vi "Main.vi"() -> ()   [LabVIEW 2019, in "Personalities Tool.lvlib"]
uses:
  Personalities Tool.lvlib
  Controls/QMH Data.ctl
  Controls/Personality Type.ctl
  Controls/roboRIO Connection Information.ctl
  Controls/Diff Key.ctl
  subVIs/Message Queue/Enqueue Message (Single).vi
panel:
  out "Personality":string
  out "Status":string
  in  "File editor":string
  in  "Download personality to RIO":bool
  in  "Save personality locally":bool
  in  "Connect":bool
  in  "Open local personality":bool
  in  "Stop":bool
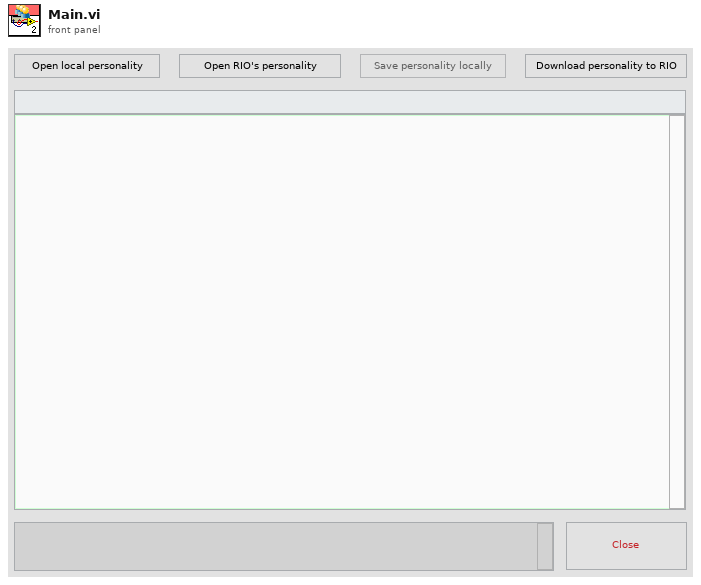
[diagram p1: front panel]
types:
  T1 = typedef "Personalities Tool.lvlib/QMH Data.ctl" = cluster{"Status":string, "Open Personality File Path":path, "File text":string, "Selected Personality":T2, "roboRIO Connection Information":T3, "VI reference":refnum<vi>, "Save personality locally reference":refnum<vi>, "File editor reference":refnum<vi>}
  T2 = typedef "Personalities Tool.lvlib/Personality Type.ctl" = cluster{"Valid personality?":bool, "Personality":string}
  T3 = typedef "Personalities Tool.lvlib/roboRIO Connection Information.ctl" = cluster{"Connected?":bool, "IP Address":string, "SN":string, "Personality":T2, "Name":string}
  T4 = typedef "Personalities Tool.lvlib/All Message Queues.ctl" = cluster{"UI":refnum<queue>}
  T5 = enum8{"Enabled", "Disabled", "Disabled and Grayed Out"}
  T6 = typedef "Personalities Tool.lvlib/Diff Key.ctl" = cluster{"Section":string, "Local":variant, "roboRIO":variant, "Selection":enum32{"Item 0", "Item 1"}, "Key":string}
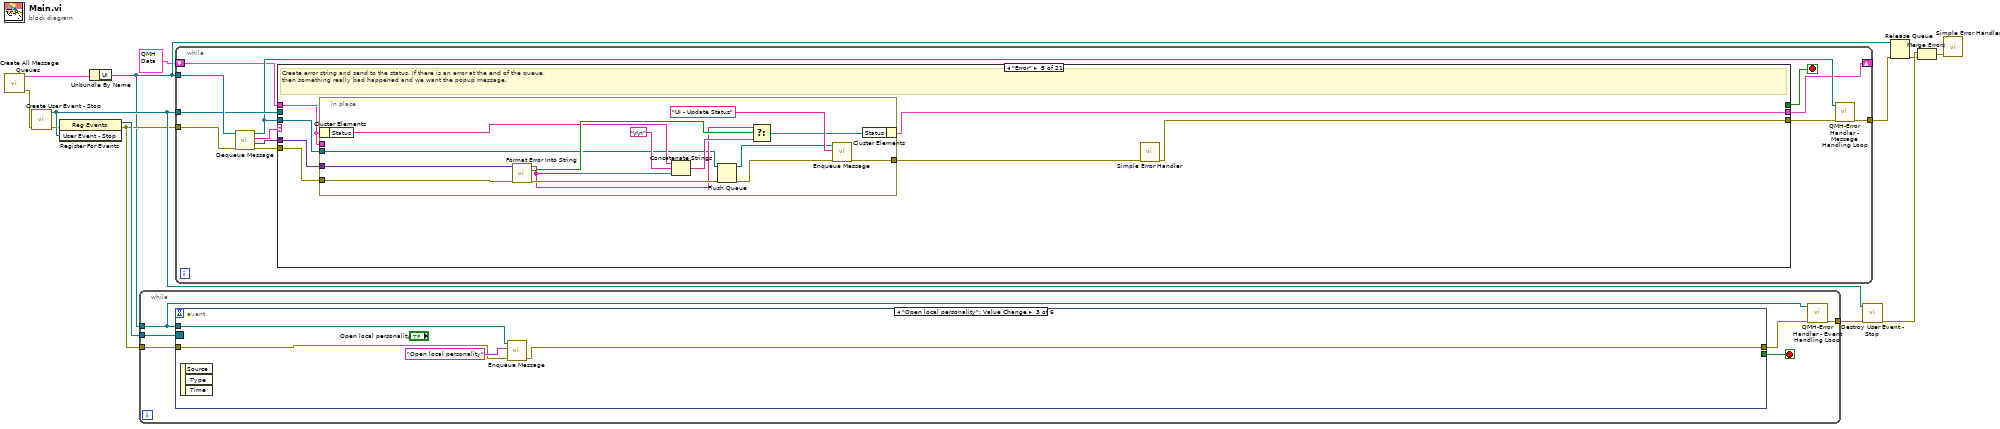
[diagram p0: block diagram]
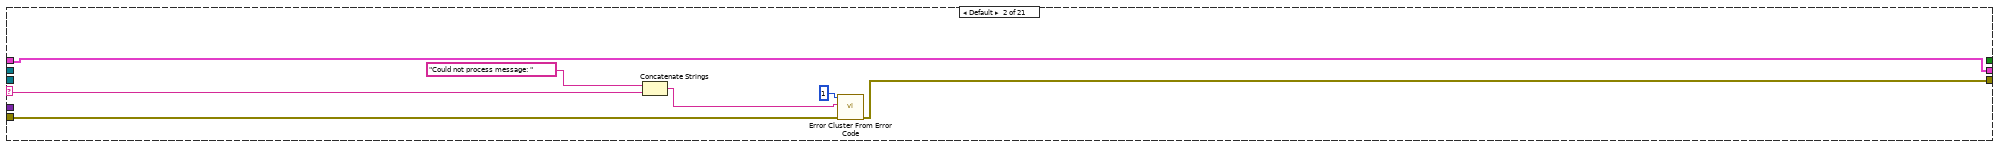
[diagram p3: hidden frame]
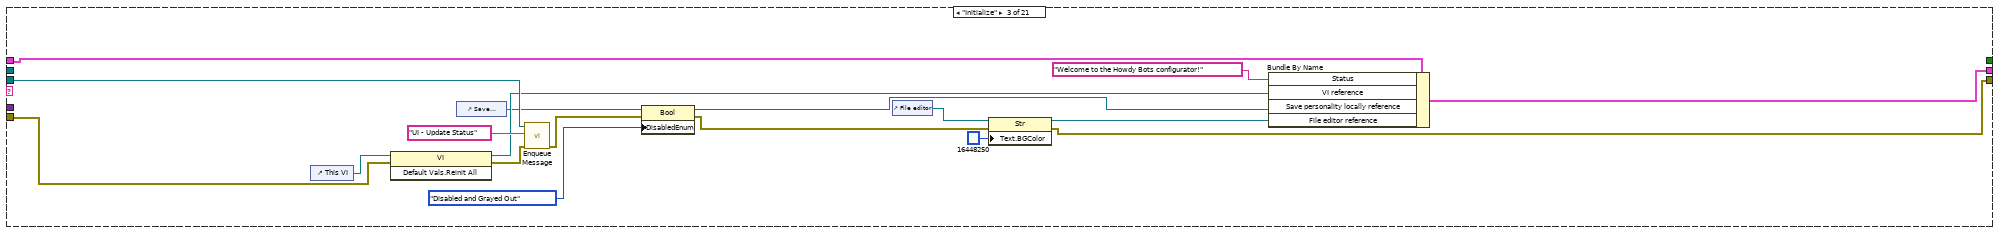
[diagram p4: hidden frame]
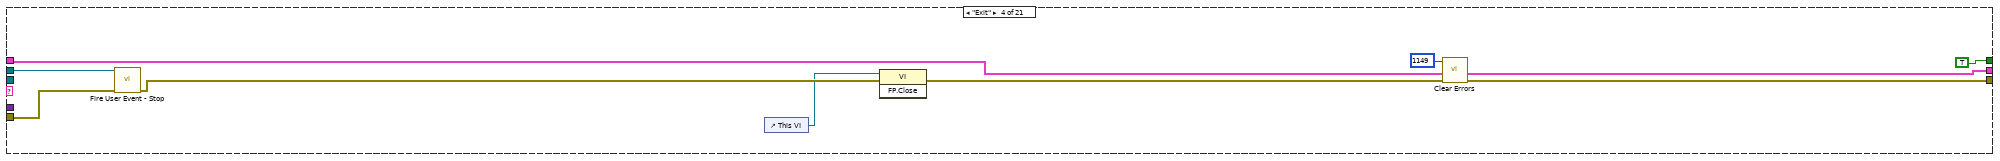
[diagram p5: hidden frame]
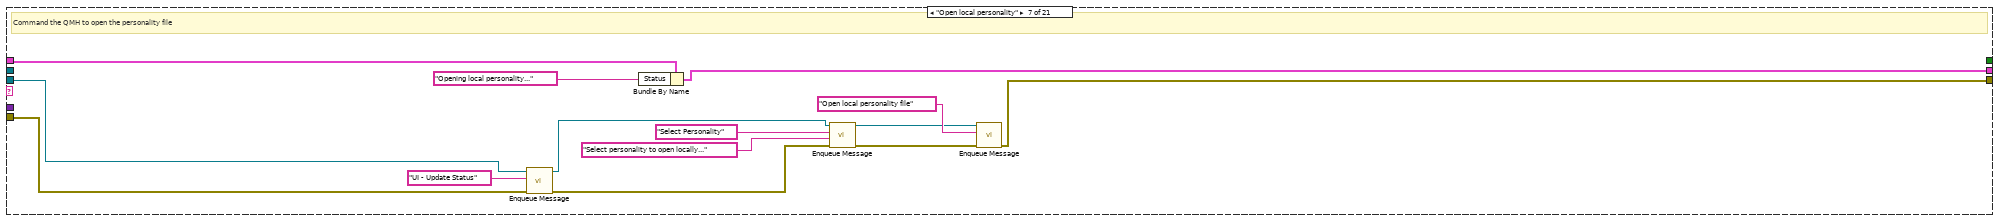
[diagram p7: hidden frame]
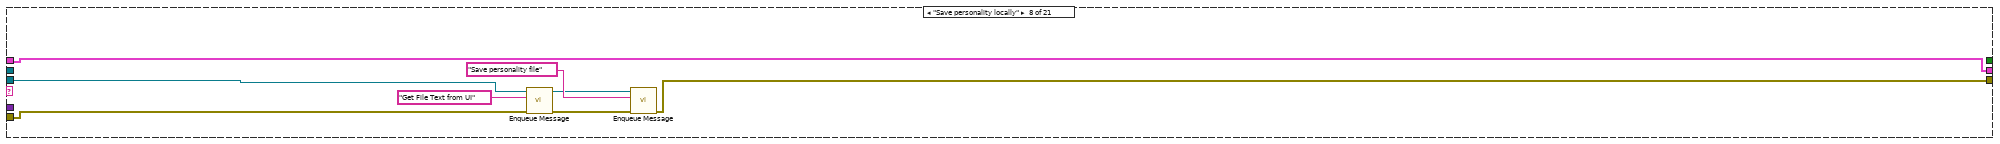
[diagram p8: hidden frame]
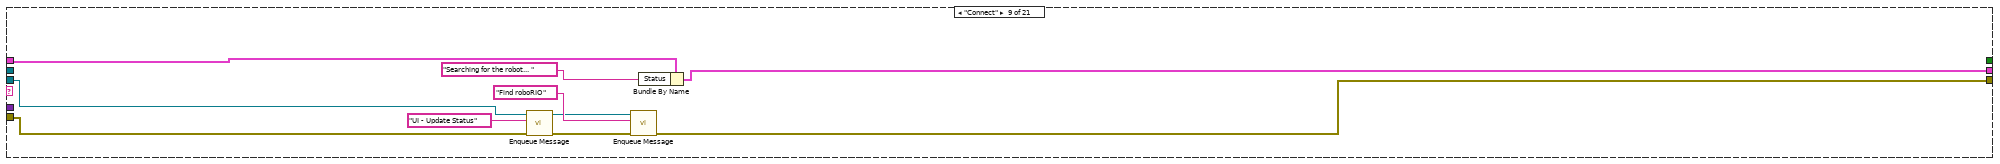
[diagram p9: hidden frame]
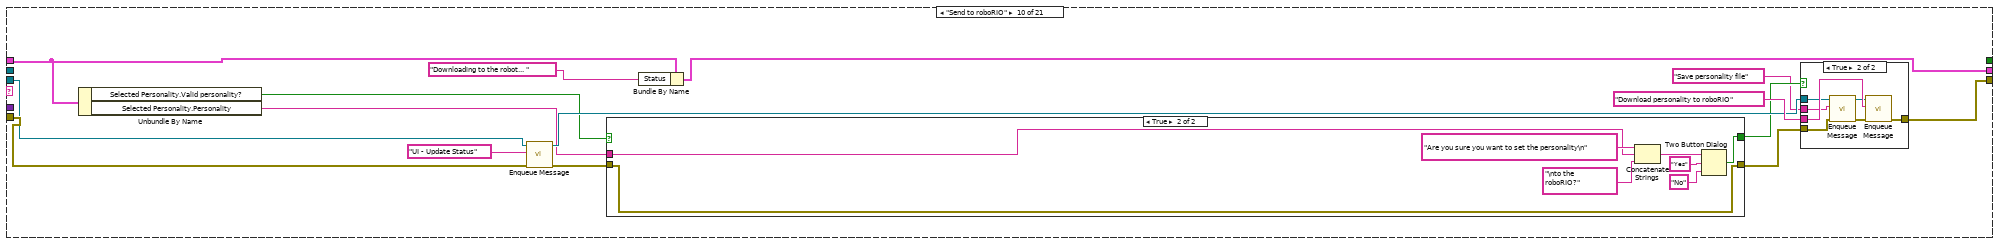
[diagram p10: hidden frame]
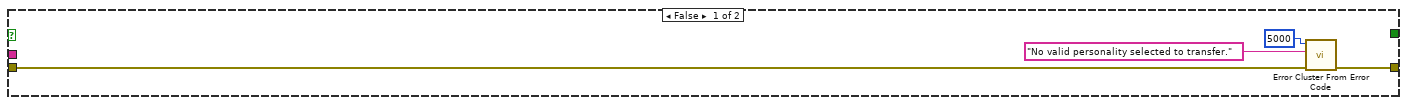
[diagram p11: hidden frame]
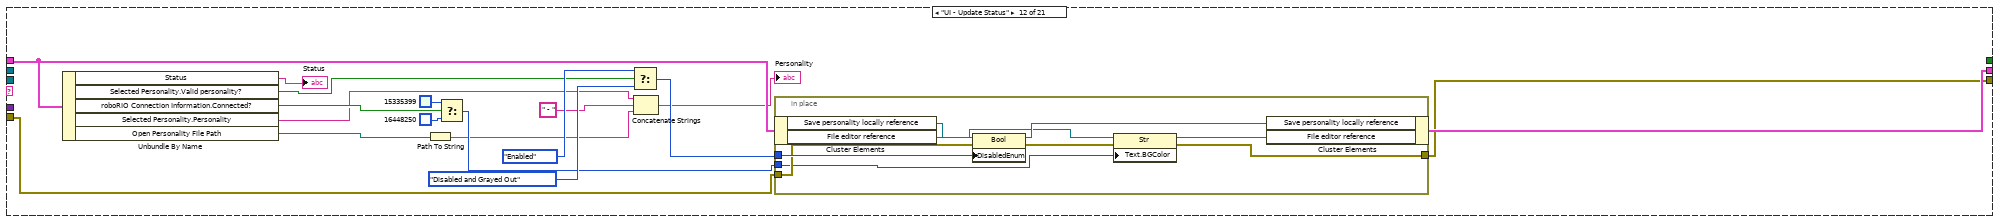
[diagram p14: hidden frame]
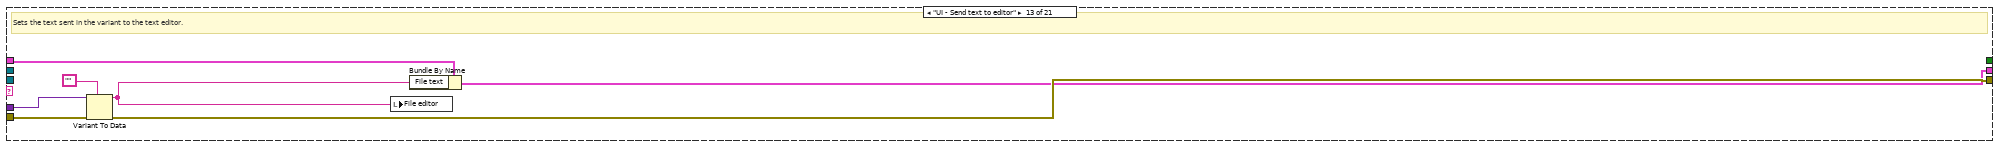
[diagram p15: hidden frame]
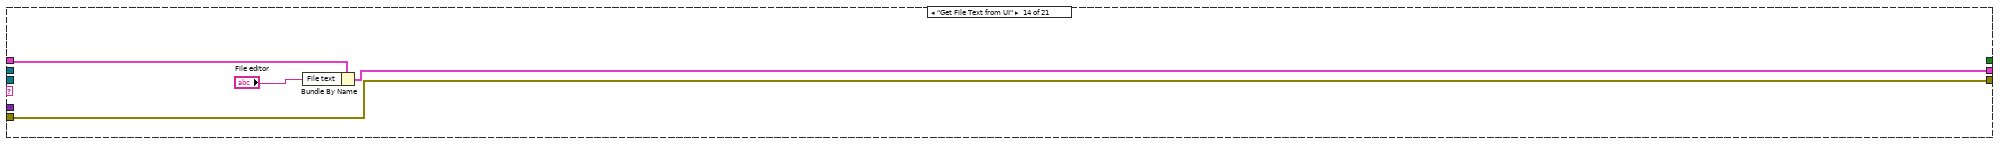
[diagram p16: hidden frame]
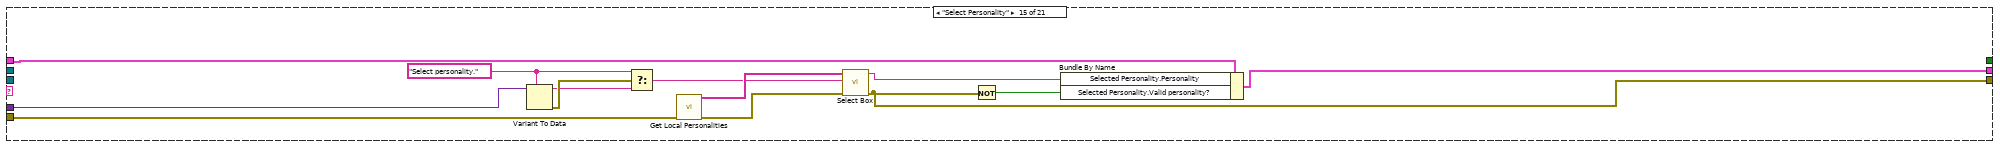
[diagram p17: hidden frame]
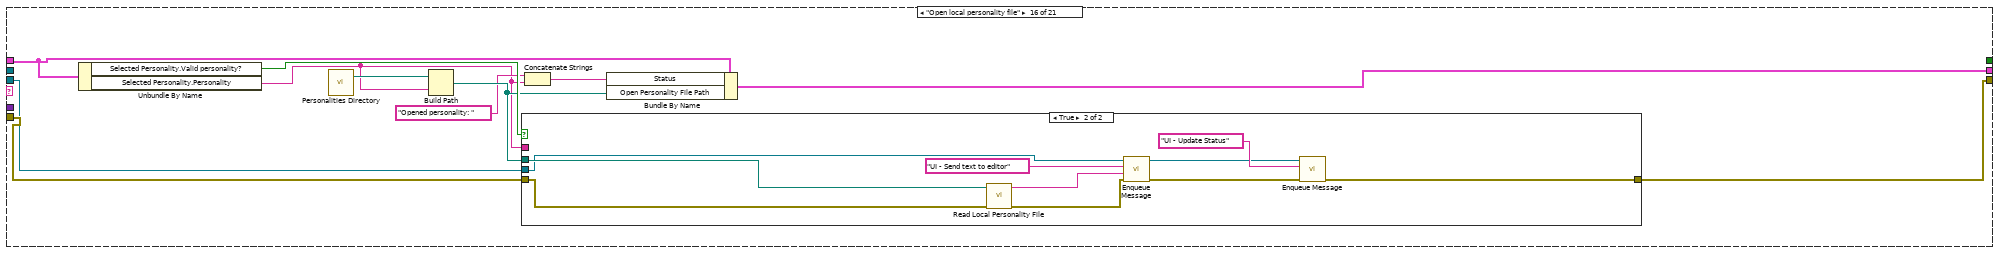
[diagram p18: hidden frame]
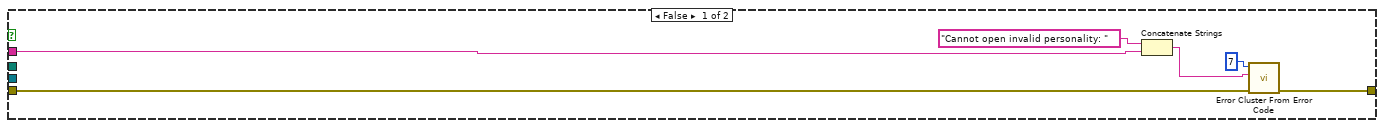
[diagram p19: hidden frame]
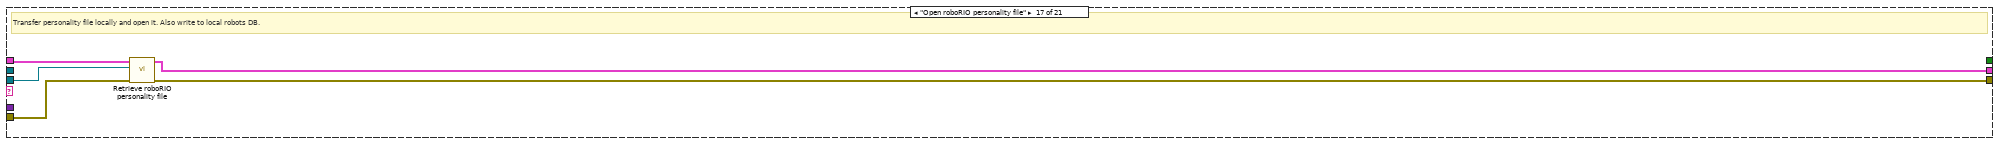
[diagram p20: hidden frame]
diagram:
  n1 = call "Create All Message Queues.vi"() -> ("error out"=w10:errorcluster, "Message Queues out"=w11:T4)  [unwired: 10 in]
  n2 = call "Create User Event - Stop.vi"("error in (no error)"=w10) -> ("error out"=w9:errorcluster, "User Event - Stop"=w12:refnum<user-event>)  [unwired: 9 in]
  n3 = register-events(error in=w9, w12) -> (reference out=w13:refnum<event-registration>, error out=w8:errorcluster)  [unwired: 1 in]
  n4 = Unbundle By Name(w11) -> ("UI"=w4:refnum<queue>)
  n5 = while {
    tunnel: w13 -> [w19]
    tunnel: w4 -> [w14]
    tunnel: w8 -> [w18]
    tunnel: [w15] -> w7
    stop <- w17 stop-if-true
    n6 = event shown="[2] \"Open local personality\": Value Change" {
      selector: w19 -> [_ _ _ _ _ _]
      dyn-events: _ -> [_ _ _ _ _ _]
      timeout: _ -> [_ _ _ _ _ _]
      tunnel: w14 -> [_ w22 w37 w41 w45 w52]
      tunnel: w18 -> [w20 w24 w39 w43 w47 w50]
      tunnel: [TRUE _ _ _ _ _] -> w17
      tunnel: [w20 w27 w38 w42 w46 w54] -> w16
      event User Event {
        n7 = event-data() -> ()  [unwired: 1 in, 3 out]
      }
      event "Stop": Value Change; Panel Close {
        n8 = event-data() -> ()  [unwired: 1 in, 3 out]
        n9 = disable-structure shown="Enabled" {
          disable-tunnel: [w28 _] -> w25
          frame Disabled {
            n10 = Two Button Dialog(message="Save opened personality before closing?", 1:"No" ("F button name (\"Cancel\")"), 2:"Yes" ("T button name (\"OK\")")) -> (T button?=w28:bool)
          }
          frame Enabled {
            # "Disabled saving check to ensure we do not accidentally override the\nfile with constants and introduce typos"
          }
        }
        n11 = case shown="True" w25 {
          tunnel: [w32 w34] -> w23
          tunnel: w24 -> [w32 w35]
          tunnel: w22 -> [_ w33]
          frame False {
          }
          frame True {
            n12 = call-poly "Enqueue Message.vi"("error in (no error)"=w35, "Message"="Save personality locally", "Message Queue"=w33) -> ("error out"=w34:errorcluster)  [unwired: 7 in, 1 out]
          }
        }
        n13 = call-poly "Enqueue Message.vi"("error in (no error)"=w23, "Message"="Exit", "Message Queue"=w22) -> ("error out"=w27:errorcluster)  [unwired: 7 in, 1 out]
      }
      event "Open local personality": Value Change {
        n14 = event-data() -> ()  [unwired: 1 in, 3 out]
        n15 = call-poly "Enqueue Message.vi"("error in (no error)"=w39, "Message"="Open local personality", "Message Queue"=w37) -> ("error out"=w38:errorcluster)  [unwired: 7 in, 1 out]
      }
      event "Connect": Value Change {
        n16 = event-data() -> ()  [unwired: 1 in, 3 out]
        n17 = call-poly "Enqueue Message.vi"("error in (no error)"=w43, "Message"="Connect", "Message Queue"=w41) -> ("error out"=w42:errorcluster)  [unwired: 7 in, 1 out]
      }
      event "Save personality locally": Value Change {
        n18 = event-data() -> ()  [unwired: 1 in, 3 out]
        n19 = call-poly "Enqueue Message.vi"("error in (no error)"=w47, "Message"="Save personality locally", "Message Queue"=w45) -> ("error out"=w46:errorcluster)  [unwired: 7 in, 1 out]
      }
      event "Download personality to RIO": Value Change {
        n20 = event-data() -> ()  [unwired: 1 in, 3 out]
        n21 = call-poly "Enqueue Message.vi"("error in (no error)"=w50, "Message"="Save personality locally", "Message Queue"=w52) -> ("error out"=w49:errorcluster, "dup Message Queue"=w51:refnum<queue>)  [unwired: 7 in]
        n22 = call-poly "Enqueue Message.vi"("error in (no error)"=w49, "Message"="Send to roboRIO", "Message Queue"=w51) -> ("error out"=w54:errorcluster)  [unwired: 7 in, 1 out]
      }
    }
    n23 = call "QMH-Error Handler - Event Handling Loop.vi"("error in (no error)"=w16, "Message Queue"=w14) -> ("dup error in"=w15:errorcluster)  [unwired: 8 in, 1 out]
  }
  n24 = while {
    tunnel: w12 -> [w60]
    tunnel: w4 -> [w67]
    tunnel: w8 -> [w66]
    tunnel: [w61] -> w5
    shift-right: [w57] -> _
    shift-left: T1 {"Status"="", "Open Personality File Path"=path "", "File text"="", "Selected Personality"={"Valid personality?"=FALSE, "Personality"=""}, "roboRIO Connection Information"={"Connected?"=FALSE, "IP Address"="", "SN"="", "Personality"={"Valid personality?"=FALSE, "Personality"=""}, "Name"=""}, "VI reference"=refnum, "Save personality locally reference"=refnum, "File editor reference"=refnum} ("UI Data") -> [w56]
    stop <- w58 stop-if-true
    n25 = call "Dequeue Message.vi"("error in (no error)"=w66, "Message Queue"=w67) -> ("error out"=w64:errorcluster, "Message Data"=w63:variant, "Message"=w65:string, "dup Message Queue"=w59:refnum<queue>)  [unwired: 6 in]
    n26 = case shown="\"Error\"" w65 {
      selector: w65 -> [_ w71 _ _ _ _ _ _ _ _ _ _ _ _ _ _ _ _ _ _ _]
      tunnel: w64 -> [w68 w76 w87 w103 w110 w125 w137 w143 w153 w170 w194 w205 w228 w232 w241 w255 w277 w287 w313 w330 w352]
      tunnel: [w68 w75 w80 w96 w106 w125 w128 w141 w151 w168 w194 w206 w227 w232 w243 w253 w278 w285 w314 w316 w349] -> w62
      tunnel: w63 -> [_ _ _ _ w109 _ _ _ _ _ _ _ w226 _ w238 _ _ _ _ _ w351]
      tunnel: w59 -> [_ _ w90 _ w108 _ w138 w142 w152 w169 _ _ _ _ _ w250 w274 w284 w311 w318 w343]
      tunnel: w60 -> [_ _ _ w102 _ _ _ _ _ _ _ _ _ _ _ _ _ _ _ _ _]
      tunnel: [_ _ _ TRUE _ _ _ _ _ _ _ _ _ _ _ _ _ _ _ _ _] -> w58
      tunnel: [w69 w70 w93 w99 w104 w126 w136 w148 w150 w167 w195 w211 w224 w231 w245 w256 w276 w288 w315 w324 w347] -> w57
      tunnel: w56 -> [w69 w70 w94 w99 w105 w126 w140 w148 w158 w164 w195 w212 w229 w233 w246 w257 w275 w289 w312 w329 w344]
      frame "---BASE QMH MESSAGES---" {
        # "This case must not execute ever, used just for documentation"
      }
      frame Default {
        n27 = Concatenate Strings("Could not process message: " ("error message (\"\")"), w71) -> (w72:string)
        n28 = call <vilib>:"Error Cluster From Error Code.vi"("error in (no error)"=w76, "error message (\"\")"=w72, "error code (0)"=1) -> ("error out"=w75:errorcluster)  [unwired: 6 in]
      }
      frame "Initialize" {
        n29 = control-ref of="This VI"() -> (w88:refnum<vi>)
        n30 = invoke class="VI" method="Default Vals.Reinit All"(reference=w88, error in=w87) -> (reference out=w85:refnum<vi>, error out=w86:errorcluster)  [unwired: 1 in, 1 out]
        n31 = control-ref of="Save personality locally"() -> (w83:refnum<vi>)
        n32 = call-poly "Enqueue Message.vi"("error in (no error)"=w86, "Message"="UI - Update Status", "Message Queue"=w90) -> ("error out"=w89:errorcluster)  [unwired: 7 in, 1 out]
        n33 = property class="Bool"(reference=w83, error in=w89, "DisabledEnum"=T5."Disabled and Grayed Out" ("Disabled")) -> (reference out=w82:refnum<vi>, error out=w84:errorcluster)
        n34 = control-ref of="File editor"() -> (w79:refnum<vi>)
        n35 = property class="Str"(reference=w79, error in=w84, "Text.BGColor"=u32 16448250 ("Text.Colors:BG Color")) -> (reference out=w78:refnum<vi>, error out=w80:errorcluster)
        n36 = Bundle By Name(cluster=w94, "Status"="Welcome to the Howdy Bots configurator!" ("element"), "VI reference"=w85, "Save personality locally reference"=w82, "File editor reference"=w78) -> (w93:T1)
      }
      frame "Exit" {
        n37 = call "Fire User Event - Stop.vi"("error in (no error)"=w103, "User Event - Stop"=w102) -> ("error out"=w101:errorcluster)  [unwired: 9 in]
        n38 = control-ref of="This VI"() -> (w97:refnum<vi>)
        n39 = invoke class="VI" method="FP.Close"(reference=w97, error in=w101) -> (error out=w98:errorcluster)  [unwired: 1 in, 2 out]
        n40 = call <vilib>:"Clear Errors.vi"("error in (no error)"=w98, "specific error code to clear (0: all)"=1149) -> ("error out"=w96:errorcluster)  [unwired: 4 in, 1 out]
      }
      frame "Error" {
        # "Create error string and send to the status. If there is an error at the end of the queue, \nthen something really bad happened and we want the popup message."
        n41 = in-place {
          in-place-border: w110 -> [w124]
          in-place-border: w109 -> [w123]
          in-place-border: w108 -> [w112]
          in-place-border: [w121] -> w107
          in-place-border: w105 -> [_]
          n42 = in-place-cluster #1(w105) -> ("Status"=w115:string)
          n43 = call "Format Error Into String.vi"("error in (no error)"=w124, "Message Data"=w123) -> ("error out"=w120:errorcluster, "error?"=w119:bool, "message"=w117:string)  [unwired: 7 in]
          n44 = Concatenate Strings(w115, "\r\n", w117) -> (w118:string)
          n45 = Flush Queue(queue=w112, error in (no error)=w120) -> (queue out=w111:refnum<queue>, error out=w113:errorcluster)  [unwired: 1 out]
          n46 = Select(t=w117, s=w119, f=w118) -> (s? t:f=w114:string)
          n47 = call-poly "Enqueue Message.vi"("error in (no error)"=w113, "Message"="UI - Update Status", "Message Queue"=w111) -> ("error out"=w121:errorcluster)  [unwired: 7 in, 1 out]
          n48 = in-place-cluster #1("Status"=w114) -> (w104:T1)
        }
        n49 = call <vilib>:"Simple Error Handler.vi"("error in (no error)"=w107) -> ("error out"=w106:errorcluster)  [unwired: 4 in, 4 out]
      }
      frame "---UI MESSAGES---" {
        # "This case must not execute ever, used just for documentation"
      }
      frame "Open local personality" {
        # "Command the QMH to open the personality file"
        n50 = call-poly "Enqueue Message.vi"("error in (no error)"=w137, "Message"="UI - Update Status", "Message Queue"=w138) -> ("error out"=w132:errorcluster, "dup Message Queue"=w133:refnum<queue>)  [unwired: 7 in]
        n51 = Bundle By Name(cluster=w140, "Status"="Opening local personality...") -> (w136:T1)
        n52 = call-poly "Enqueue Message.vi"("error in (no error)"=w132, "Message Data"="Select personality to open locally..." ("Message"), "Message"="Select Personality", "Message Queue"=w133) -> ("error out"=w129:errorcluster, "dup Message Queue"=w127:refnum<queue>)  [unwired: 6 in]
        n53 = call-poly "Enqueue Message.vi"("error in (no error)"=w129, "Message"="Open local personality file", "Message Queue"=w127) -> ("error out"=w128:errorcluster)  [unwired: 7 in, 1 out]
      }
      frame "Save personality locally" {
        n54 = call-poly "Enqueue Message.vi"("error in (no error)"=w143, "Message"="Get File Text from UI", "Message Queue"=w142) -> ("error out"=w144:errorcluster, "dup Message Queue"=w145:refnum<queue>)  [unwired: 7 in]
        n55 = call-poly "Enqueue Message.vi"("error in (no error)"=w144, "Message"="Save personality file", "Message Queue"=w145) -> ("error out"=w141:errorcluster)  [unwired: 7 in, 1 out]
      }
      frame "Connect" {
        n56 = call-poly "Enqueue Message.vi"("error in (no error)"=w153, "Message"="UI - Update Status", "Message Queue"=w152) -> ("error out"=w154:errorcluster, "dup Message Queue"=w155:refnum<queue>)  [unwired: 7 in]
        n57 = call-poly "Enqueue Message.vi"("error in (no error)"=w154, "Message"="Find roboRIO", "Message Queue"=w155) -> ("error out"=w151:errorcluster)  [unwired: 7 in, 1 out]
        n58 = Bundle By Name(cluster=w158, "Status"="Searching for the robot... ") -> (w150:T1)
      }
      frame "Send to roboRIO" {
        n59 = Unbundle By Name(w164) -> ("Selected Personality.Valid personality?"=w162:bool, "Selected Personality.Personality"=w163:string)
        n60 = call-poly "Enqueue Message.vi"("error in (no error)"=w170, "Message"="UI - Update Status", "Message Queue"=w169) -> ("error out"=w161:errorcluster, "dup Message Queue"=w171:refnum<queue>)  [unwired: 7 in]
        n61 = case shown="True" w162 {
          tunnel: [_ w182] -> w165
          tunnel: w163 -> [_ w179]
          tunnel: [w176 w178] -> w160
          tunnel: w161 -> [w177 w178]
          frame False {
            n62 = call <vilib>:"Error Cluster From Error Code.vi"("error in (no error)"=w177, "error message (\"\")"="No valid personality selected to transfer." ("error message (\"\")"), "error code (0)"=5000) -> ("error out"=w176:errorcluster)  [unwired: 6 in]
          }
          frame True {
            n63 = Concatenate Strings("Are you sure you want to set the personality\n" ("message"), w179, "\nto the roboRIO?" ("message")) -> (w181:string)
            n64 = Two Button Dialog(message=w181, 1:"No" ("F button name (\"Cancel\")"), 2:"Yes" ("T button name (\"OK\")")) -> (T button?=w182:bool)
          }
        }
        n65 = Bundle By Name(cluster=w164, "Status"="Downloading to the robot... ") -> (w167:T1)
        n66 = case shown="True" w165 {
          tunnel: "Download personality to roboRIO" ("Message") -> [_ w193]
          tunnel: w171 -> [_ w189]
          tunnel: w160 -> [w186 w192]
          tunnel: [w186 w190] -> w168
          tunnel: "Save personality file" ("Message") -> [_ w187]
          frame False {
          }
          frame True {
            n67 = call-poly "Enqueue Message.vi"("error in (no error)"=w192, "Message"=w187, "Message Queue"=w189) -> ("error out"=w191:errorcluster, "dup Message Queue"=w188:refnum<queue>)  [unwired: 7 in]
            n68 = call-poly "Enqueue Message.vi"("error in (no error)"=w191, "Message"=w193, "Message Queue"=w188) -> ("error out"=w190:errorcluster)  [unwired: 7 in, 1 out]
          }
        }
      }
      frame "---SUPPORT FUNCTIONS---" {
        # "This case must not execute ever, used just for documentation"
      }
      frame "UI - Update Status" {
        n69 = Unbundle By Name(w212) -> ("Status"=→"Status":string, "Selected Personality.Valid personality?"=w208:bool, "roboRIO Connection Information.Connected?"=w204:bool, "Selected Personality.Personality"=w199:string, "Open Personality File Path"=w200:path)
        n70 = Path To String(path=w200) -> (string=w198:string)
        n71 = Select(t=u32 15335399 ("Text.Colors:FG Color"), s=w204, f=u32 16448250 ("Text.Colors:BG Color")) -> (s? t:f=w203:u32)
        n72 = Select(t=T5."Enabled" ("Disabled"), s=w208, f=T5."Disabled and Grayed Out" ("Disabled")) -> (s? t:f=w209:T5)
        n73 = Concatenate Strings(w199, " - " ("string"), w198) -> (→"Personality":string)
        n74 = in-place {
          in-place-border: w209 -> [w222]
          in-place-border: w205 -> [w219]
          in-place-border: [w215] -> w206
          in-place-border: w203 -> [w214]
          n75 = in-place-cluster #2(w212) -> ("Save personality locally reference"=w221:refnum<vi>, "File editor reference"=w218:refnum<vi>)
          n76 = property class="Bool"(reference=w221, error in=w219, "DisabledEnum"=w222) -> (reference out=w220:refnum<vi>, error out=w216:errorcluster)
          n77 = property class="Str"(reference=w218, error in=w216, "Text.BGColor"=w214) -> (reference out=w217:refnum<vi>, error out=w215:errorcluster)
          n78 = in-place-cluster #2("Save personality locally reference"=w220, "File editor reference"=w217) -> (w211:T1)
        }
      }
      frame "UI - Send text to editor" {
        # "Sets the text sent in the variant to the text editor."
        n79 = Variant To Data(error in=w228, type="", Variant=w226) -> (data=w223:string, error out=w227:errorcluster)
        n80 = local write "File editor"(w223) -> ()
        n81 = Bundle By Name(cluster=w229, "File text"=w223) -> (w224:T1)
      }
      frame "Get File Text from UI" {
        n82 = Bundle By Name(cluster=w233, "File text"="File editor") -> (w231:T1)
      }
      frame "Select Personality" {
        w236 = "Select personality."
        n83 = Variant To Data(type=w236, Variant=w238) -> (data=w235:string, error out=w237:errorcluster)  [unwired: 1 in]
        n84 = Select(t=w236, s=w237, f=w235) -> (s? t:f=w234:string)
        n85 = call "Get Local Personalities.vi"("error in (no error)"=w241) -> ("error out"=w240:errorcluster, "Personalities"=w239:string[])  [unwired: 9 in]
        n86 = call "Select Box.vi"("error in (no error)"=w240, "UI message"=w234, "Selections available"=w239) -> ("error out"=w243:errorcluster, "Selection"=w244:string)  [unwired: 7 in]
        n87 = Not(x=w243) -> (.not. x?=w242:bool)
        n88 = Bundle By Name(cluster=w246, "Selected Personality.Personality"=w244, "Selected Personality.Valid personality?"=w242) -> (w245:T1)
      }
      frame "Open local personality file" {
        n89 = Unbundle By Name(w257) -> ("Selected Personality.Valid personality?"=w254:bool, "Selected Personality.Personality"=w247:string)
        n90 = call "Personalities Directory.vi"() -> ("appended path"=w252:path)  [unwired: 3 in]
        n91 = Build Path(base path=w252, name or relative path=w247) -> (appended path=w251:path)
        n92 = case shown="True" w254 {
          tunnel: w255 -> [w263 w273]
          tunnel: w247 -> [w258 _]
          tunnel: [w262 w264] -> w253
          tunnel: w251 -> [_ w272]
          tunnel: w250 -> [_ w269]
          frame False {
            n93 = Concatenate Strings("Cannot open invalid personality: " ("error message (\"\")"), w258) -> (w259:string)
            n94 = call <vilib>:"Error Cluster From Error Code.vi"("error in (no error)"=w263, "error message (\"\")"=w259, "error code (0)"=7) -> ("error out"=w262:errorcluster)  [unwired: 6 in]
          }
          frame True {
            n95 = call "Read Local Personality File.vi"("error in (no error)"=w273, "File Path"=w272) -> ("error out"=w270:errorcluster, "Personality text"=w268:string)  [unwired: 7 in, 1 out]
            n96 = call-poly "Enqueue Message.vi"("error in (no error)"=w270, "Message Data"=w268, "Message"="UI - Send text to editor", "Message Queue"=w269) -> ("error out"=w265:errorcluster, "dup Message Queue"=w266:refnum<queue>)  [unwired: 6 in]
            n97 = call-poly "Enqueue Message.vi"("error in (no error)"=w265, "Message"="UI - Update Status", "Message Queue"=w266) -> ("error out"=w264:errorcluster)  [unwired: 7 in, 1 out]
          }
        }
        n98 = Concatenate Strings("Opened personality: " ("Status"), w247) -> (w248:string)
        n99 = Bundle By Name(cluster=w257, "Status"=w248, "Open Personality File Path"=w251) -> (w256:T1)
      }
      frame "Open roboRIO personality file" {
        # "Transfer personality file locally and open it. Also write to local robots DB."
        n100 = call "Retrieve roboRIO personality file.vi"("error in (no error)"=w277, "Message Queue"=w274, "UI Data Out"=w275) -> ("error out"=w278:errorcluster, "UI Data in"=w276:T1)  [unwired: 7 in]
      }
      frame "Save personality file" {
        n101 = Unbundle By Name(w289) -> ("Selected Personality.Valid personality?"=w286:bool, "Selected Personality.Personality"=w283:string, "Open Personality File Path"=w282:path, "File text"=w281:string)
        n102 = case shown="False" w286 {
          tunnel: w287 -> [w296 w307]
          tunnel: w283 -> [w293 w299]
          tunnel: [w295 w298] -> w285
          tunnel: w282 -> [w290 w308]
          tunnel: w284 -> [_ w310]
          tunnel: [w291 w300] -> w280
          tunnel: w281 -> [_ w301]
          tunnel: [w290 w297] -> w279
          frame False {
            n103 = Concatenate Strings("Cannot save invalid personality: " ("error message (\"\")"), w293) -> (w291:string)
            n104 = call <vilib>:"Error Cluster From Error Code.vi"("error in (no error)"=w296, "error message (\"\")"=w291, "error code (0)"=7) -> ("error out"=w295:errorcluster)  [unwired: 6 in]
          }
          frame True {
            n105 = call "Save Local Personality File.vi"("error in (no error)"=w307, "New Content"=w301, "File Path"=w308) -> ("error out"=w302:errorcluster, "Path out"=w297:path)  [unwired: 7 in]
            n106 = call-poly "Enqueue Message.vi"("Message"="UI - Update Status", "Message Queue"=w310) -> ("error out"=w303:errorcluster)  [unwired: 8 in, 1 out]
            n107 = Merge Errors(w302, w303) -> (w298:errorcluster)
            n108 = Select(t="Could not save personality: ", s=w298, f="Saved personality: " ("Status")) -> (s? t:f=w306:string)
            n109 = Concatenate Strings(w306, w299) -> (w300:string)
          }
        }
        n110 = Bundle By Name(cluster=w289, "Open Personality File Path"=w279, "Status"=w280) -> (w288:T1)
      }
      frame "Find roboRIO" {
        n111 = call "Find roboRIO.vi"("error in (no error)"=w313, "Queue In"=w311, "UI Data in"=w312) -> ("error out"=w314:errorcluster, "UI Data out"=w315:T1)  [unwired: 7 in]
      }
      frame "Download personality to roboRIO" {
        # "#TODO"
        n112 = Unbundle By Name(w329) -> ("Open Personality File Path"=w320:path, "roboRIO Connection Information"=w328:T3)
        n113 = call "Transfer file to roboRIO.vi"("error in (no error)"=w330, "roboRIO Connection Information in"=w328, "Configuration File Path"=w320) -> ("error out"=w327:errorcluster, "roboRIO Connection Information out"=w326:T3, "Status"=w325:string)  [unwired: 6 in]
        n114 = case shown="Error" w327 {
          selector: w327 -> [w333 _]
          tunnel: [w333 w337] -> w322
          tunnel: [w332 w335] -> w321
          tunnel: w326 -> [w332 _]
          tunnel: [w331 w336] -> w323
          tunnel: w325 -> [w331 _]
          tunnel: w320 -> [_ w334]
          frame No Error {
          }
          frame Error {
            # "If we are already connected, \nwe try that connection the first time.\nIf we fail, then we query for roboRIOs again"
            n115 = call "Transfer file to roboRIO.vi"("Configuration File Path"=w334) -> ("error out"=w337:errorcluster, "roboRIO Connection Information out"=w335:T3, "Status"=w336:string)  [unwired: 8 in]
          }
        }
        n116 = Bundle By Name(cluster=w329, "Status"=w323, "roboRIO Connection Information"=w321) -> (w324:T1)
        n117 = call "Set Personality with SN.vi"("error in (no error)"=w322, "roboRIO Connection Information"=w321) -> ("error out"=w317:errorcluster)  [unwired: 9 in]
        n118 = call-poly "Enqueue Message.vi"("error in (no error)"=w317, "Message"="UI - Update Status", "Message Queue"=w318) -> ("error out"=w316:errorcluster)  [unwired: 7 in, 1 out]
      }
      frame "Diff" {
        n119 = Bundle("Diff conflicts"=T6[] [], path[] []) -> (w341:cluster{"Diff conflicts":T6[], path[]})  [unwired: 1 in]
        n120 = Variant To Data(error in=w352, type=w341, Variant=w351) -> (data=w348:cluster{"Diff conflicts":T6[], path[]}, error out=w350:errorcluster)
        n121 = Unbundle(w348) -> ("Diff conflicts"=w338:T6[], w340:path[])
        n122 = Index Array(array=w340) -> (element #1=w345:path, element #2=w346:path)  [unwired: 2 in]
        n123 = call "Diff Tool.vi"("Diff conflicts"=w338, "Message Queue"=w343, "error in (no error)"=w350, "roboRIO"=w346, "Local"=w345, "UI Data in"=w344) -> ("error out"=w349:errorcluster, "UI Data out"=w347:T1)  [unwired: 4 in]
      }
    }
    n124 = call "QMH-Error Handler - Message Handling Loop.vi"("error in (no error)"=w62, "Message Queue"=w59) -> ("dup error in"=w61:errorcluster)  [unwired: 8 in, 1 out]
  }
  n125 = call "Destroy User Event - Stop.vi"("error in (no error)"=w7, "User Event - Stop"=w12) -> ("error out"=w6:errorcluster)  [unwired: 9 in]
  n126 = Release Queue(queue=w4, error in (no error)=w5) -> (error out=w3:errorcluster)  [unwired: 1 in, 2 out]
  n127 = Merge Errors(w6, w3) -> (w2:errorcluster)
  n128 = call <vilib>:"Simple Error Handler.vi"("error in (no error)"=w2) -> ()  [unwired: 4 in, 5 out]
